vi "input.vi"(8 "error in":errorcluster, 10 "data table in":T1, 11 "Tagbus PID Module runtime in":refnum<class "Tagbus PID Module runtime.lvclass">) -> (0 "error out":errorcluster, 2 "data table out":T1, 3 "Tagbus PID Module runtime out":refnum<class "Tagbus PID Module runtime.lvclass">)   [LabVIEW 2014, in "Tagbus PID Module runtime.lvclass"]
doc: "Provides an interface for reading data from a module at runtime. While this interface performs no operations, a child should provide an override which may read from any open sessions, references, or interfaces."
uses:
  Tagbus PID Module runtime.lvclass
  <vilib>/NI/Tag Bus/table/data table.ctl
  Tagbus PID Module runtime.lvclass/Tagbus PID Module runtime.ctl
  <vilib>/NI/Tag Bus/table/data polymorphs/write many/write Doubles.vi
  <vilib>/NI/Tag Bus/table/data table.lvlib
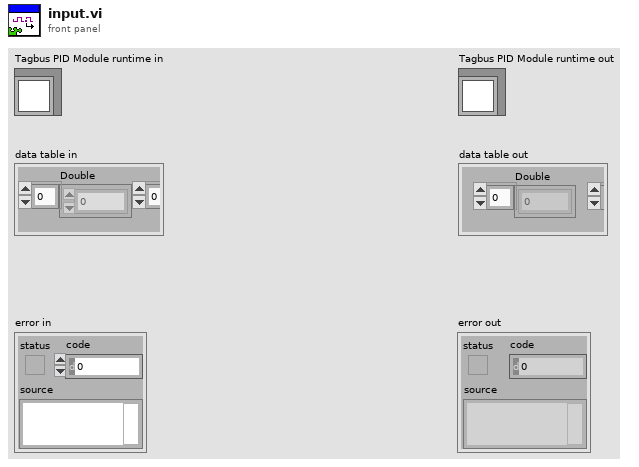
[diagram p1: front panel]
types:
  T1 = typedef "tag bus.lvlib/data table.lvlib/data table.ctl" = cluster{"Double":dbl[], "Single":sgl[], "I64":i64[], "I32":i32[], "I16":i16[], "I8":i8[], "U64":u64[], "U32":u32[], "U16":u16[], "U8":u8[], "Boolean":bool[], "String":string[], "Array of Double":cluster{"DBL Array":dbl[]}[], "Array of Single":cluster{"SGL Array":sgl[]}[], "Array of I64":cluster{"I64 Array":i64[]}[], "Array of I32":cluster{"I32 Array":i32[]}[], "Array of I16":cluster{"I16 Array":i16[]}[], "Array of I8":cluster{"I8 Array":i8[]}[], "Array of U64":cluster{"U64 Array":u64[]}[], "Array of U32":cluster{"U32 Array":u32[]}[], "Array of U16":cluster{"U16 Array":u16[]}[], "Array of U8":cluster{"U8 Array":u8[]}[], "Array of Boolean":cluster{"Boolean Array":bool[]}[], "Array of String":cluster{"String Array":string[]}[]}
  T2 = cluster{"control indices":i32[], "data indices":i32[]}[]
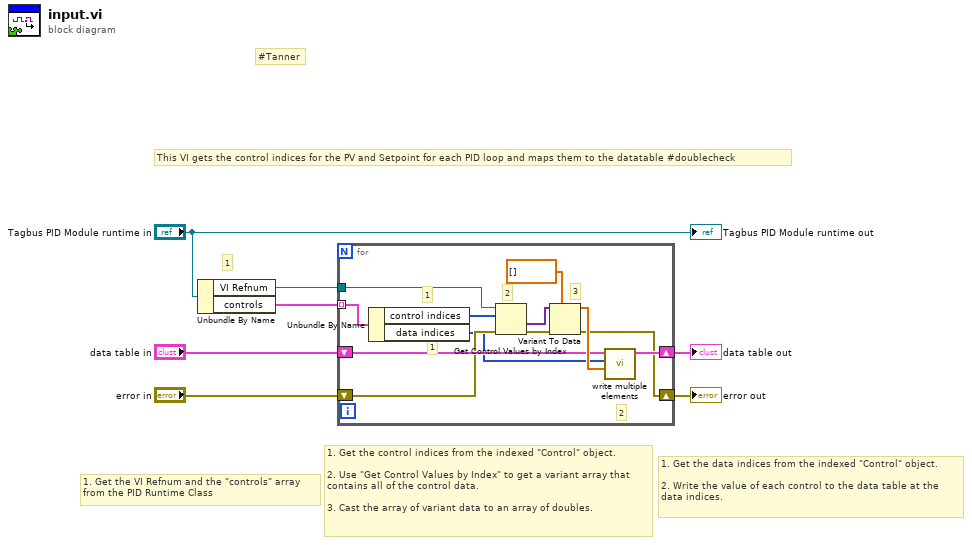
[diagram p0: block diagram]
diagram:
  # "#Tanner"
  # "This VI gets the control indices for the PV and Setpoint for each PID loop and maps them to the datatable #doublecheck"
  # "1. Get the data indices from the indexed \"Control\" object.\n\n2. Write the value of each control to the data table at the \ndata indices."
  # "1. Get the control indices from the indexed \"Control\" object.\n\n2. Use \"Get Control Values by Index\" to get a variant array that\ncontains all of the control data.\n\n3. Cast the array of variant data to an array of doubles."
  # "1"
  # "1. Get the VI Refnum and the \"controls\" array\nfrom the PID Runtime Class"
  n1 = Unbundle By Name("Tagbus PID Module runtime in") -> ("VI Refnum"=w1:refnum<vi>, "controls"=w7:T2)
  n2 = for {
    tunnel: w7 -> [w19] mode=indexing
    shift-right: [w11] -> w5
    shift-left: "error in" -> [w12]
    shift-right: [w14] -> w2
    shift-left: "data table in" -> [w15]
    tunnel: w1 -> [w8]
    # "2"
    # "1"
    # "3"
    # "2"
    # "1"
    n3 = Unbundle By Name(w19) -> ("control indices"=w10:i32[], "data indices"=w9:i32[])
    n4 = Get Control Values by Index(0:w8, 1:w10, 3:w12) -> (10:w18:variant[], 11:w13:errorcluster)
    n5 = Variant To Data(error in=w13, type=dbl[] [], Variant=w18) -> (data=w16:dbl[], error out=w11:errorcluster)
    n6 = call-poly <vilib>:"write multiple elements.vi"("values"=w16, "indices"=w9, "data table in"=w15) -> ("data table out"=w14:T1)  [unwired: 8 in]
  }
  "error out" <- w5
  "data table out" <- w2
  "Tagbus PID Module runtime out" <- "Tagbus PID Module runtime in"
